vi "Setup Position.vi"(0 "error in (no error)":errorcluster) -> (1 "function return":i32, 2 "error out":errorcluster)   [LabVIEW 2014, in "MCM3000.lvlib"]
doc: "long SetupPosition();"
uses:
  MCM3000.lvlib
  ThorMCM3000.dll
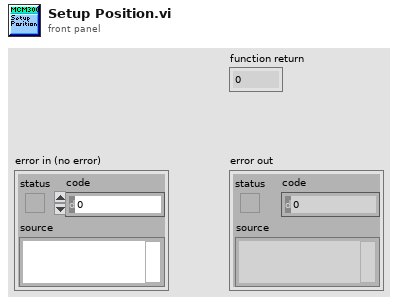
[diagram p1: front panel]
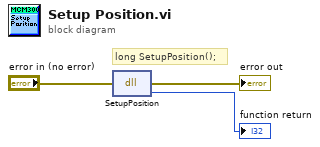
[diagram p0: block diagram]
diagram:
  # "long SetupPosition();"
  n1 = dll-call lib="C:/TIS_CalebVS2012/TIS_Development/Hardware/SDKs/MCM3000_SDK/LabVIEW/inc/ThorMCM3000.*" fn="SetupPosition"(error in="error in (no error)") -> (error out=→"error out":errorcluster, →"function return":i32)  [unwired: 2 in, 1 out]
